vi "GDSLvIcon_CreatePictureWord.vi"(1 "Word":string, 5 "error in (no error)":errorcluster) -> (15 "WordData":T1, 19 "error out":errorcluster)   [LabVIEW 2014]
doc: "Creates a picture word."
uses:
  <resource>/Framework/Providers/Open_GDS/ClassProviders/Common/LvIcon_class/subvis/GDSLvIcon_WordDataType.ctl
panel:
  out "Picture(Compressed)":bool[][](array[boolean])
  out "Picture(Normal)":bool[][](array[boolean])
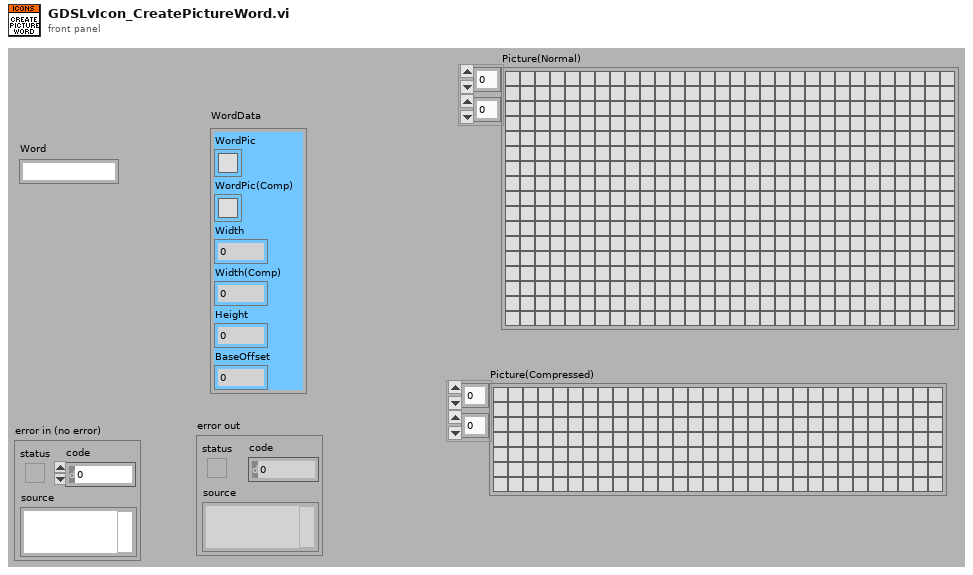
[diagram p1: front panel]
types:
  T1 = typedef "GDSLvIcon_WordDataType.ctl" = cluster{"WordPic":bool[][], "WordPic(Comp)":bool[][], "Width":i32, "Width(Comp)":i32, "Height":i32, "BaseOffset":i32}
  T2 = cluster{"CharPattern":bool[][], "CharPattern(Compressed)":bool[][], i8}
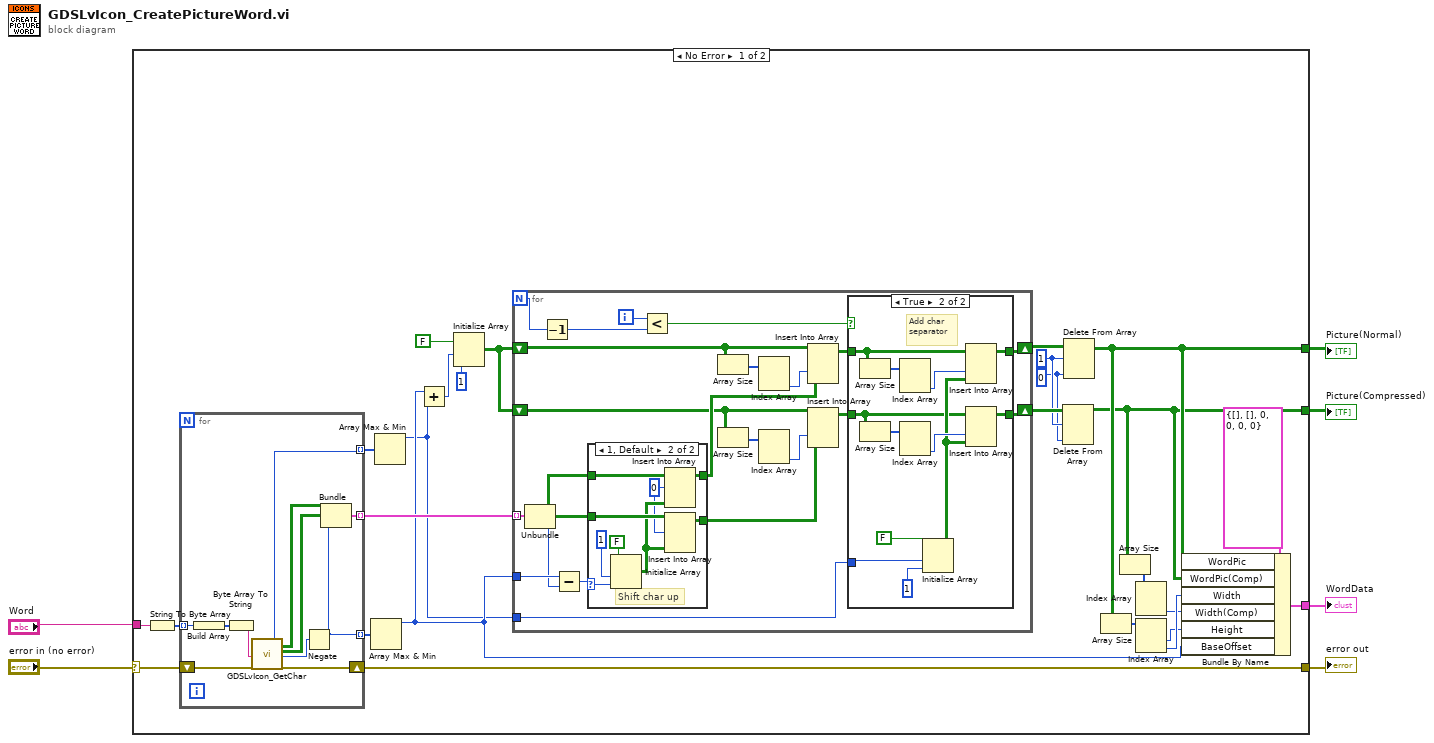
[diagram p0: block diagram]
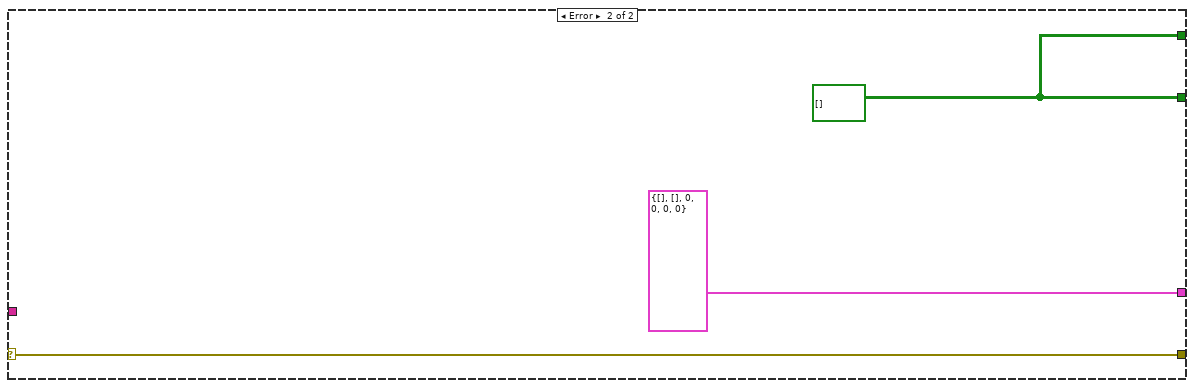
[diagram p4: hidden frame]
diagram:
  n1 = case shown="No Error" "error in (no error)" {
    selector: "error in (no error)" -> [w13 w94]
    tunnel: [w14 w94] -> w5
    tunnel: "Word" -> [w29 _]
    tunnel: [w11 w93] -> w1
    tunnel: [w31 T1 {"WordPic"=[], "WordPic(Comp)"=[], "Width"=0, "Width(Comp)"=0, "Height"=0, "BaseOffset"=0} ("WordData")] -> w3
    tunnel: [w9 w93] -> w2
    frame No Error {
      w7 = 0
      w8 = 1
      n2 = String To Byte Array(string=w29) -> (unsigned byte array=w30:u8[])
      n3 = for {
        tunnel: w30 -> [w90] mode=indexing
        tunnel: [w88] -> w28 mode=indexing
        tunnel: [w87] -> w27 mode=indexing
        tunnel: [w83] -> w21 mode=indexing
        shift-right: [w81] -> w14
        shift-left: w13 -> [w82]
        n4 = Build Array(w90) -> (w91:u8[])
        n5 = Byte Array To String(unsigned byte array=w91) -> (string=w89:string)
        n6 = call <resource>:"GDSLvIcon_GetChar.vi"("Char"=w89, "error in (no error)"=w82) -> ("CharHeight"=w83:i8, "CharPattern"=w85:bool[][], "CharPattern(Compressed)"=w84:bool[][], "Base Offset Out"=w86:i8, "error out"=w81:errorcluster)  [unwired: 13 in]
        n7 = Negate(x=w86) -> (-x=w87:i8)
        n8 = Bundle("CharPattern"=w85, "CharPattern(Compressed)"=w84, w87) -> (w88:T2)  [unwired: 1 in]
      }
      n9 = Array Max & Min(array=w27) -> (max value=w18:i8)  [unwired: 3 out]
      n10 = Array Max & Min(array=w21) -> (max value=w16:i8)  [unwired: 3 out]
      n11 = Add(x=w18, y=w16) -> (x+y=w19:i8)
      n12 = Initialize Array(FALSE, w19, 1 ("Numeric")) -> (w20:bool[][])
      n13 = for {
        N -> [w54]
        tunnel: w28 -> [w33] mode=indexing
        shift-right: [w41] -> w12
        shift-left: w20 -> [w45]
        tunnel: w18 -> [w51]
        shift-right: [w35] -> w10
        shift-left: w20 -> [w38]
        tunnel: w16 -> [w34]
        i -> [w53]
        n14 = Unbundle(w33) -> ("CharPattern"=w48:bool[][], "CharPattern(Compressed)"=w47:bool[][], w50:i8)
        n15 = Decrement(x=w54) -> (x-1=w55:i32)
        n16 = Subtract(x=w51, y=w50) -> (x-y=w49:i8)
        n17 = case shown="1, Default" w49 {
          selector: w49 -> [_ w60]
          tunnel: w48 -> [w57 w66]
          tunnel: w47 -> [w56 w65]
          tunnel: [w57 w64] -> w43
          tunnel: [w56 w63] -> w37
          frame 0 {
          }
          frame 1, Default {
            w59 = 0 ("Index (row)")
            # "Shift char up"
            n18 = Initialize Array(FALSE, 1 ("Numeric"), w60) -> (w62:bool[][])
            n19 = Insert Into Array(array=w66, index (row)=w59, new element=w62) -> (w64:bool[][])  [unwired: 1 in]
            n20 = Insert Into Array(array=w65, index (row)=w59, new element=w62) -> (w63:bool[][])  [unwired: 1 in]
          }
        }
        n21 = Less?(x=w53, y=w55) -> (x < y?=w52:bool)
        n22 = Array Size(array=w45) -> (size(s)=w46:i32[])
        n23 = Array Size(array=w38) -> (size(s)=w39:i32[])
        n24 = Index Array(array=w46) -> (element #2=w44:i32)  [unwired: 2 in, 1 out]
        n25 = Index Array(array=w39) -> (element #2=w40:i32)  [unwired: 2 in, 1 out]
        n26 = Insert Into Array(array=w45, index (col)=w44, new element=w43) -> (w42:bool[][])  [unwired: 1 in]
        n27 = Insert Into Array(array=w38, index (col)=w40, new element=w37) -> (w36:bool[][])  [unwired: 1 in]
        n28 = case shown="True" w52 {
          tunnel: w42 -> [w68 w79]
          tunnel: [w68 w80] -> w41
          tunnel: w36 -> [w67 w72]
          tunnel: [w67 w74] -> w35
          tunnel: w34 -> [_ w70]
          frame False {
          }
          frame True {
            # "Add char\nseparator"
            n29 = Array Size(array=w79) -> (size(s)=w78:i32[])
            n30 = Array Size(array=w72) -> (size(s)=w75:i32[])
            n31 = Index Array(array=w78) -> (element #2=w77:i32)  [unwired: 2 in, 1 out]
            n32 = Index Array(array=w75) -> (element #2=w76:i32)  [unwired: 2 in, 1 out]
            n33 = Initialize Array(FALSE, w70, 1 ("Dimension Size")) -> (w73:bool[][])
            n34 = Insert Into Array(array=w79, index (col)=w77, new element=w73) -> (w80:bool[][])  [unwired: 1 in]
            n35 = Insert Into Array(array=w72, index (col)=w76, new element=w73) -> (w74:bool[][])  [unwired: 1 in]
          }
        }
      }
      n36 = Delete From Array(array=w10, length=w8, index (col)=w7) -> (array with subset deleted=w9:bool[][])  [unwired: 1 in, 1 out]
      n37 = Delete From Array(array=w12, length=w8, index (col)=w7) -> (array with subset deleted=w11:bool[][])  [unwired: 1 in, 1 out]
      n38 = Array Size(array=w11) -> (size(s)=w26:i32[])
      n39 = Array Size(array=w9) -> (size(s)=w23:i32[])
      n40 = Index Array(array=w23) -> (element #2=w24:i32)  [unwired: 2 in, 1 out]
      n41 = Index Array(array=w26) -> (element #1=w22:i32, element #2=w25:i32)  [unwired: 2 in]
      n42 = Bundle By Name(cluster=T1 {"WordPic"=[], "WordPic(Comp)"=[], "Width"=0, "Width(Comp)"=0, "Height"=0, "BaseOffset"=0} ("WordData"), "WordPic"=w11, "WordPic(Comp)"=w9, "Width"=w25, "Width(Comp)"=w24, "Height"=w22, "BaseOffset"=w18) -> (w31:T1)
    }
    frame Error {
      w93 = bool[][] []
    }
  }
  "error out" <- w5
  "Picture(Normal)" <- w1
  "WordData" <- w3
  "Picture(Compressed)" <- w2
